vi "Lockstep Stop.vi"(8 "error in (no error)":errorcluster, 9 "Device Number":string, 10 "Lockstep Group (1)":u8=1, 11 "VISA resource name":refnum<visa-resource-name>) -> (0 "error out":errorcluster, 3 "VISA resource name out":refnum<visa-resource-name>)   [LabVIEW 2013, in "Zaber A Series.lvlib"]
doc: "Halts a lockstep motion already in progress. This command must be used to halt the motion of a lockstep group created with the Enable Lockstep VI; the normal stop command will not work.\n\nThis VI requires that the Initialize VI has been called with the same serial port, and that the specified lockstep group has been enabled."
uses:
  Zaber A Series.lvlib
  Private/All Commands.ctl
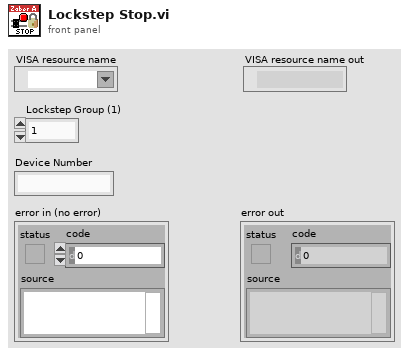
[diagram p1: front panel]
types:
  T1 = typedef "Zaber A Series.lvlib/All Commands.ctl" = string
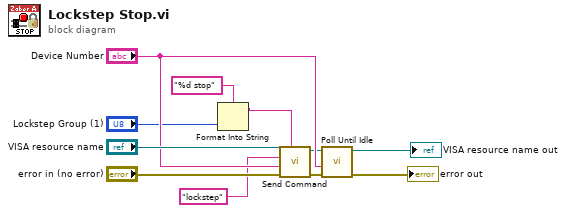
[diagram p0: block diagram]
diagram:
  n1 = Format Into String(format string="%d stop", "Lockstep Group (1)") -> (resulting string=w4:string)  [unwired: 2 in, 1 out]
  n2 = call "Send Command.vi"("Data"=w4, "error in (no error)"="error in (no error)", "Device and Axis"="Device Number", "Command"=T1 "lockstep" ("Complete Command List"), "VISA resource name"="VISA resource name") -> ("error out"=w8:errorcluster, "VISA resource name out"=w7:refnum<visa-resource-name>)  [unwired: 1 in, 4 out]
  n3 = call "Poll Until Idle.vi"("error in (no error)"=w8, "Device and Axis"="Device Number", "VISA resource name"=w7) -> ("error out"=→"error out":errorcluster, "VISA resource name out"=→"VISA resource name out":refnum<visa-resource-name>)  [unwired: 7 in]
